vi "扫描脚本.vi"(1 "4-wire":bool, 2 "扫描":T1 {"测试参数"."反向极限电流(mA)" min=0.0 max=3000.0; "测试参数"."反向电压(V)" min=0.0 max=40.0; "测试参数"."电压改变量(V)" min=0.0 max=40.0 step=5e-06; "测试参数"."正向极限电流(mA)" min=0.0 max=3000.0; "测试参数"."正向电压(V)" min=0.0 max=40.0}, 3 "方向(T:正向)":bool=TRUE) -> (0 "Script":string)   [LabVIEW 2021]
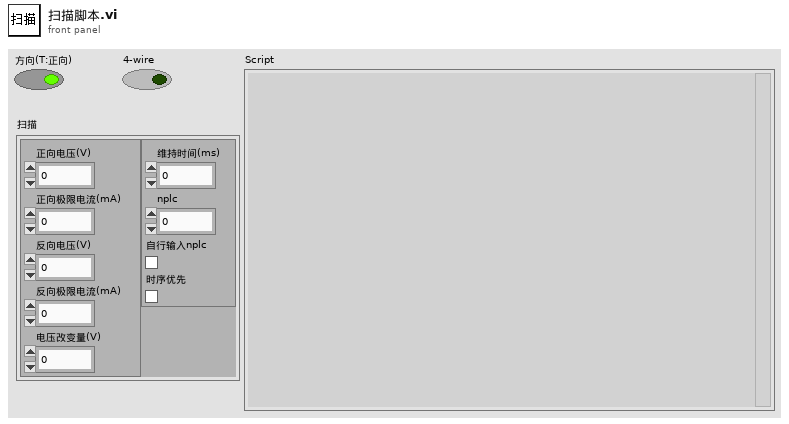
[diagram p1: front panel]
types:
  T1 = typedef "扫描参数.ctl" = cluster{"测试参数":cluster{"正向电压(V)":dbl, "正向极限电流(mA)":dbl, "反向电压(V)":dbl, "反向极限电流(mA)":dbl, "电压改变量(V)":dbl}, "时序参数":cluster{"维持时间(ms)":dbl, "nplc":dbl, "自行输入nplc":bool, "时序优先":bool}}
  T2 = cluster{"正向电压(V)":dbl, "正向极限电流(mA)":dbl, "反向电压(V)":dbl, "反向极限电流(mA)":dbl, "电压改变量(V)":dbl}
  T3 = cluster{"维持时间(ms)":dbl, "nplc":dbl, "自行输入nplc":bool, "时序优先":bool}
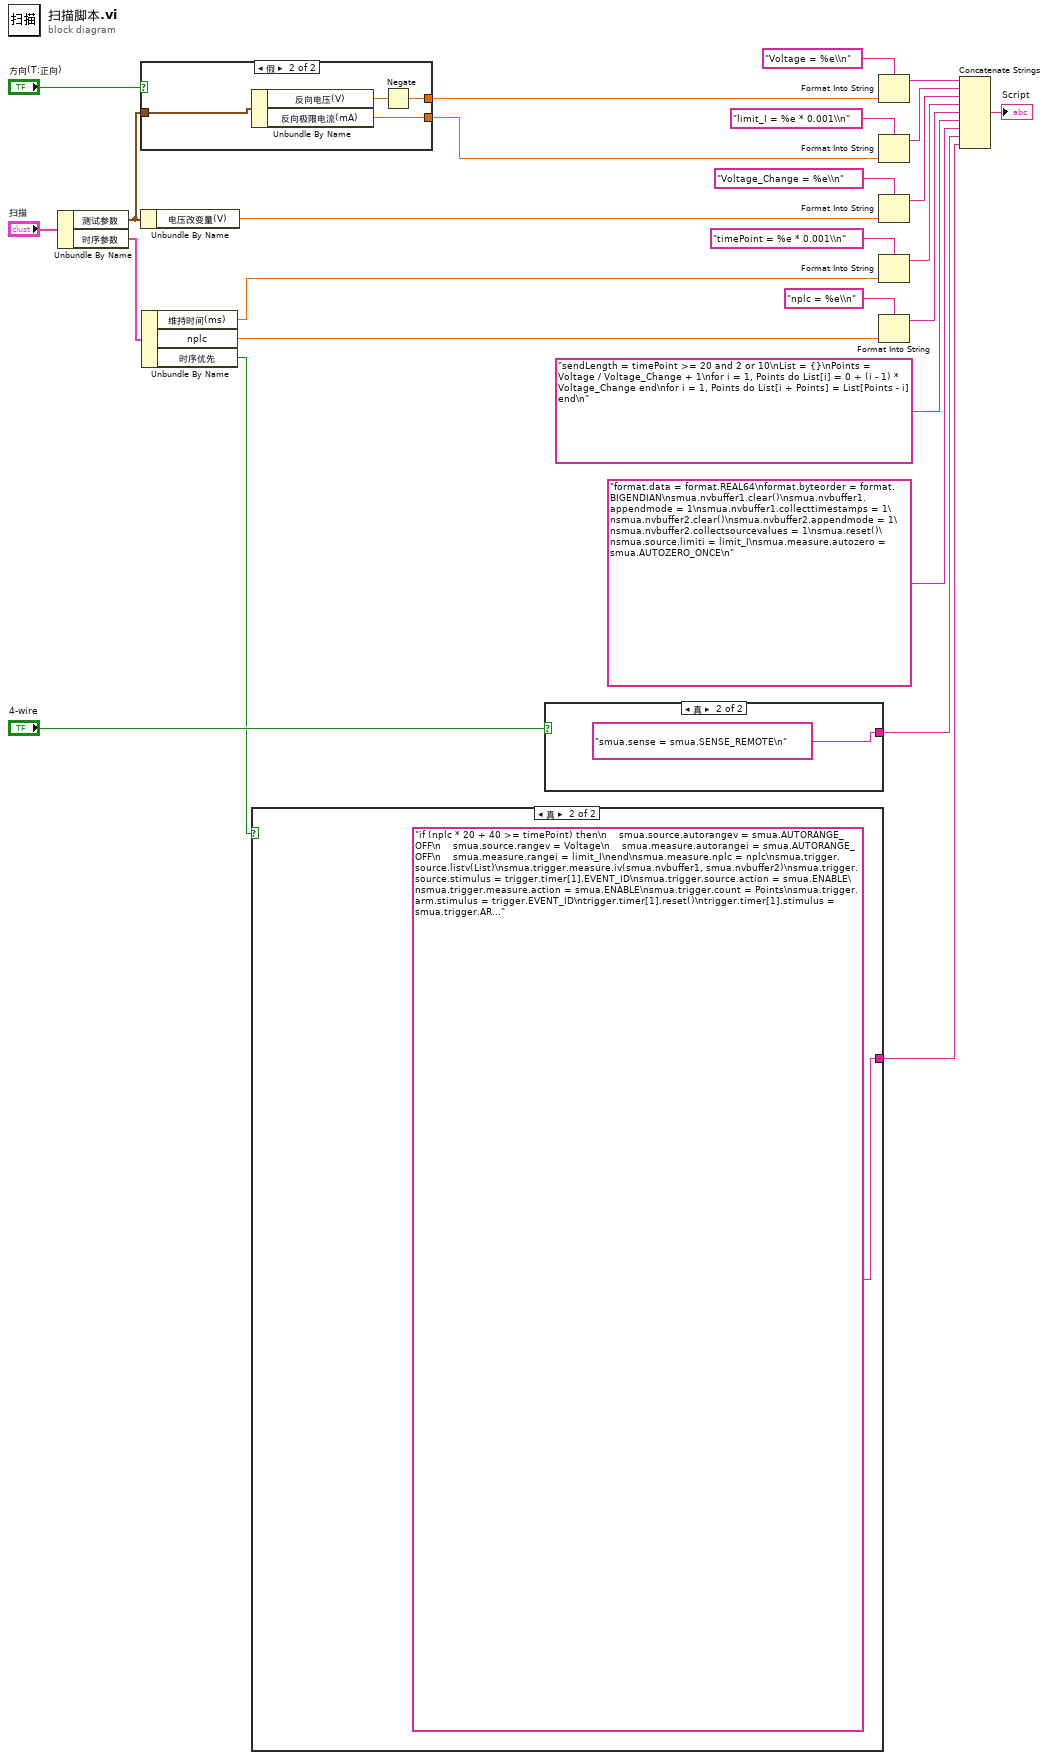
[diagram p0: block diagram]
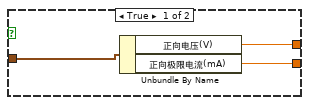
[diagram p2: hidden frame]
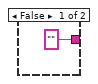
[diagram p3: hidden frame]
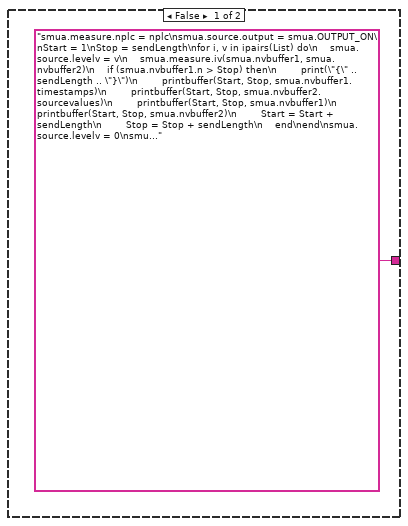
[diagram p4: hidden frame]
diagram:
  n1 = Unbundle By Name("扫描") -> ("测试参数"=w11:T2, "时序参数"=w14:T3)
  n2 = case shown="假" "方向(T:正向)" {
    tunnel: w11 -> [w29 w33]
    tunnel: [w28 w30] -> w9
    tunnel: [w27 w32] -> w6
    frame True {
      n3 = Unbundle By Name(w29) -> ("正向电压(V)"=w28:dbl, "正向极限电流(mA)"=w27:dbl)
    }
    frame False {
      n4 = Unbundle By Name(w33) -> ("反向电压(V)"=w31:dbl, "反向极限电流(mA)"=w32:dbl)
      n5 = Negate(x=w31) -> (-x=w30:dbl)
    }
  }
  n6 = Unbundle By Name(w11) -> ("电压改变量(V)"=w12:dbl)
  n7 = Unbundle By Name(w14) -> ("维持时间(ms)"=w2:dbl, "nplc"=w5:dbl, "时序优先"=w1:bool)
  n8 = case shown="真" w1 {
    tunnel: ["smua.measure.nplc = nplc\nsmua.source.output = smua.OUTPUT_ON\nStart = 1\nStop = sendLength\nfor i, v in ipairs(List) do\n    smua.source.levelv = v\n    smua.measure.iv(smua.nvbuffer1, smua.nvbuffer2)\n    if (smua.nvbuffer1.n > Stop) then\n        print(\"{\" .. sendLength .. \"}\")\n        printbuffer(Start, Stop, smua.nvbuffer1.timestamps)\n        printbuffer(Start, Stop, smua.nvbuffer2.sourcevalues)\n        printbuffer(Start, Stop, smua.nvbuffer1)\n        printbuffer(Start, Stop, smua.nvbuffer2)\n        Start = Start + sendLength\n        Stop = Stop + sendLength\n    end\nend\nsmua.source.levelv = 0\nsmua.source.output = smua.OUTPUT_OFF\nStop = Points\nprint(\"{\" .. Stop - Start + 1 .. \"}\")\nprintbuffer(Start, Stop, smua.nvbuffer1.timestamps)\nprintbuffer(Start, Stop, smua.nvbuffer2.sourcevalues)\nprintbuffer(Start, Stop, smua.nvbuffer1)\nprintbuffer(Start, Stop, smua.nvbuffer2)\nprint(\"{done}\")\nreset()" "if (nplc * 20 + 40 >= timePoint) then\n    smua.source.autorangev = smua.AUTORANGE_OFF\n    smua.source.rangev = Voltage\n    smua.measure.autorangei = smua.AUTORANGE_OFF\n    smua.measure.rangei = limit_I\nend\nsmua.measure.nplc = nplc\nsmua.trigger.source.listv(List)\nsmua.trigger.measure.iv(smua.nvbuffer1, smua.nvbuffer2)\nsmua.trigger.source.stimulus = trigger.timer[1].EVENT_ID\nsmua.trigger.source.action = smua.ENABLE\nsmua.trigger.measure.action = smua.ENABLE\nsmua.trigger.count = Points\nsmua.trigger.arm.stimulus = trigger.EVENT_ID\ntrigger.timer[1].reset()\ntrigger.timer[1].stimulus = smua.trigger.ARMED_EVENT_ID\ntrigger.timer[1].passthrough = false\ntrigger.timer[1].delay = timePoint\ntrigger.timer[1].count = Points\nsmua.source.output = smua.OUTPUT_ON\nsmua.trigger.initiate()\ndelay(1e-3)\nsmua.trigger.arm.set()\nfunction _done()\n    Start = 1\n    Stop = sendLength\n    repeat\n        if (bit.test(status.operation.instrument.smua.condition, 4) == false) then\n            smua.source.leveli = 0\n            smua.source.levelv = 0\n            smua.source.output = smua.OUTPUT_OFF\n            Stop = Points\n            print(\"{\" .. Stop - Start + 1 .. \"}\")\n            printbuffer(Start, Stop, smua.nvbuffer1.timestamps)\n            printbuffer(Start, Stop, smua.nvbuffer2.sourcevalues)\n            printbuffer(Start, Stop, smua.nvbuffer1)\n            printbuffer(Start, Stop, smua.nvbuffer2)\n            print(\"{done}\")\n            return\n        elseif (smua.nvbuffer1.n > Stop) then\n            print(\"{\" .. sendLength .. \"}\")\n            printbuffer(Start, Stop, smua.nvbuffer1.timestamps)\n            printbuffer(Start, Stop, smua.nvbuffer2.sourcevalues)\n            printbuffer(Start, Stop, smua.nvbuffer1)\n            printbuffer(Start, Stop, smua.nvbuffer2)\n            Start = Start + sendLength\n            Stop = Stop + sendLength\n        end\n        delay(timePoint)\n    until (false)\nend\n_done()\nreset()"] -> w18
    frame False {
    }
    frame True {
    }
  }
  n9 = case shown="真" "4-wire" {
    tunnel: ["" "smua.sense = smua.SENSE_REMOTE\n"] -> w17
    frame False {
    }
    frame True {
    }
  }
  n10 = Format Into String(format string="Voltage = %e\\n" ("格式字符串"), w9) -> (resulting string=w23:string)  [unwired: 2 in, 1 out]
  n11 = Format Into String(format string="limit_I = %e * 0.001\\n" ("格式字符串"), w6) -> (resulting string=w7:string)  [unwired: 2 in, 1 out]
  n12 = Format Into String(format string="Voltage_Change = %e\\n" ("格式字符串"), w12) -> (resulting string=w8:string)  [unwired: 2 in, 1 out]
  n13 = Format Into String(format string="timePoint = %e * 0.001\\n", w2) -> (resulting string=w4:string)  [unwired: 2 in, 1 out]
  n14 = Format Into String(format string="nplc = %e\\n", w5) -> (resulting string=w3:string)  [unwired: 2 in, 1 out]
  n15 = Concatenate Strings(w23, w7, w8, w4, w3, "sendLength = timePoint >= 20 and 2 or 10\nList = {}\nPoints = Voltage / Voltage_Change + 1\nfor i = 1, Points do List[i] = 0 + (i - 1) * Voltage_Change end\nfor i = 1, Points do List[i + Points] = List[Points - i] end\n", "format.data = format.REAL64\nformat.byteorder = format.BIGENDIAN\nsmua.nvbuffer1.clear()\nsmua.nvbuffer1.appendmode = 1\nsmua.nvbuffer1.collecttimestamps = 1\nsmua.nvbuffer2.clear()\nsmua.nvbuffer2.appendmode = 1\nsmua.nvbuffer2.collectsourcevalues = 1\nsmua.reset()\nsmua.source.limiti = limit_I\nsmua.measure.autozero = smua.AUTOZERO_ONCE\n", w17, w18) -> (→"Script":string)
